vi "Release Msg Q DVR.vi"(10 "Msg Q DVR":refnum<data-value>) -> (0 "error out":errorcluster)   [LabVIEW 2021, in "jettl.lvlib"]
uses:
  jettl.lvlib
  Msg/Msg.lvclass
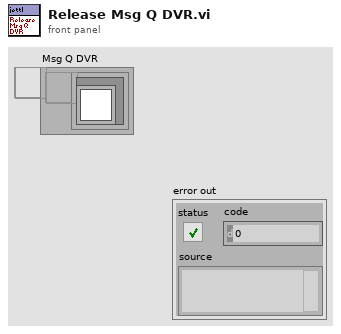
[diagram p1: front panel]
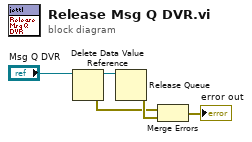
[diagram p0: block diagram]
diagram:
  n1 = Delete Data Value Reference(data value reference="Msg Q DVR") -> (data value=w5:refnum<queue>, error out=w1:errorcluster)  [unwired: 1 in]
  n2 = Release Queue(queue=w5) -> (error out=w3:errorcluster)  [unwired: 2 in, 2 out]
  n3 = Merge Errors(w1, w3) -> (→"error out":errorcluster)
